vi "探头窗口-24-4列-网络版.vi"() -> ()   [LabVIEW 2017]
panel:
  in  "外部停止命令？":bool=TRUE
  out "引用-监测模式？":refnum<vi>
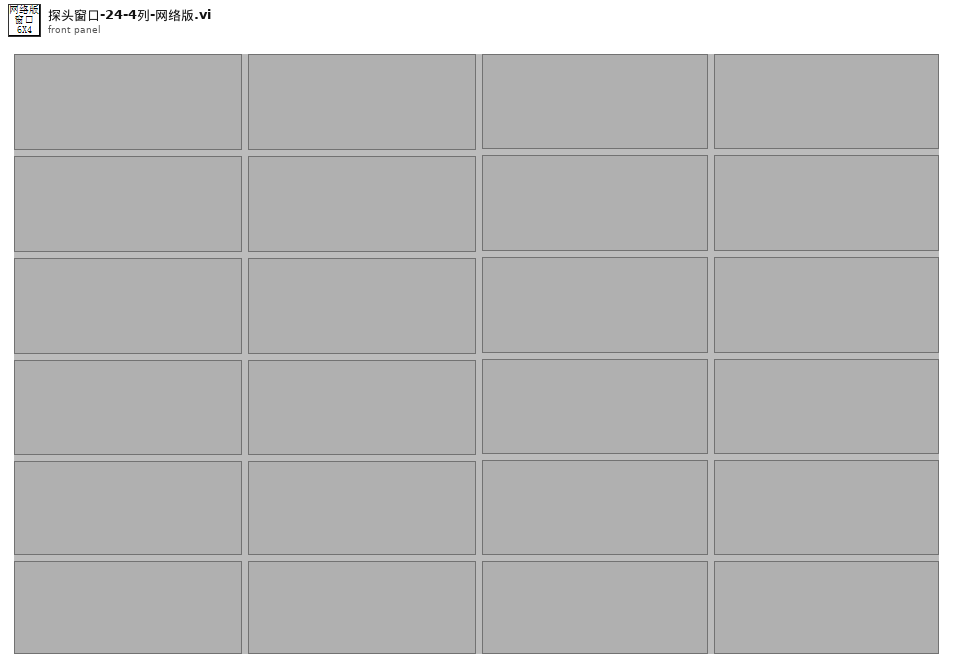
[diagram p1: front panel]
types:
  T1 = typedef "eventvkey.ctl" = enum16{"ASCII", "Enter", "Return", "Shift", "Ctrl", "Alt", "Cmd", "Opt", "Caps", "NumLock", "Clear", "Break", "Up", "Down", "Left", "Right", "Insert", "Delete", "Home", "End", "PageUp", "PageDown", "Escape", "Help", "Pause", "ScrollLock", "F1", "F2", "F3", "F4", "F5", "F6", "F7", "F8", "F9", "F10", "F11", "F12", "F13", "F14", "F15", "F16", "F17", "F18", "F19", "F20", "F21", "F22", "F23", "F24", "Play", "VolumeUp", "VolumeDown", "Mute", "Two Byte Char"}
  T2 = typedef "探头属性.ctl" = cluster{"探头地址与信息":T3, "测量值":T6, "限值":T7, "探头状态":T8, "累积记录":T9, "报警方式":T10}
  T3 = typedef "探测器信息.ctl" = cluster{"网络地址":string, "名称":string, "备注":string, "累积剂量":dbl, "累积限值":dbl, "硬件剂量率限值":T4, "剂量率限值1":dbl, "剂量率限值2":dbl, "报警方式":T5}
  T4 = typedef "探头剂量率限值选择.ctl" = enum16{"一级限值", "二级限值"}
  T5 = typedef "报警方式选择.ctl" = enum16{"常报警", "自动静音", "手动静音"}
  T6 = typedef "测量值.ctl" = cluster{"时间":timestamp, "数值":dbl}
  T7 = typedef "剂量率限值.ctl" = cluster{"限值1":dbl, "限值2":dbl, "探头限值":T4}
  T8 = typedef "探头状态.ctl" = enum16{"正常", "离线", "禁用", "一级报警", "二级报警", "累积报警"}
  T9 = typedef "单条累积记录.ctl" = cluster{"起始时间":timestamp, "结束时间":timestamp, "累积剂量":dbl}
  T10 = typedef "报警方式.ctl" = cluster{"报警方式":T5, "延迟计时":u16, "报警中？":bool}
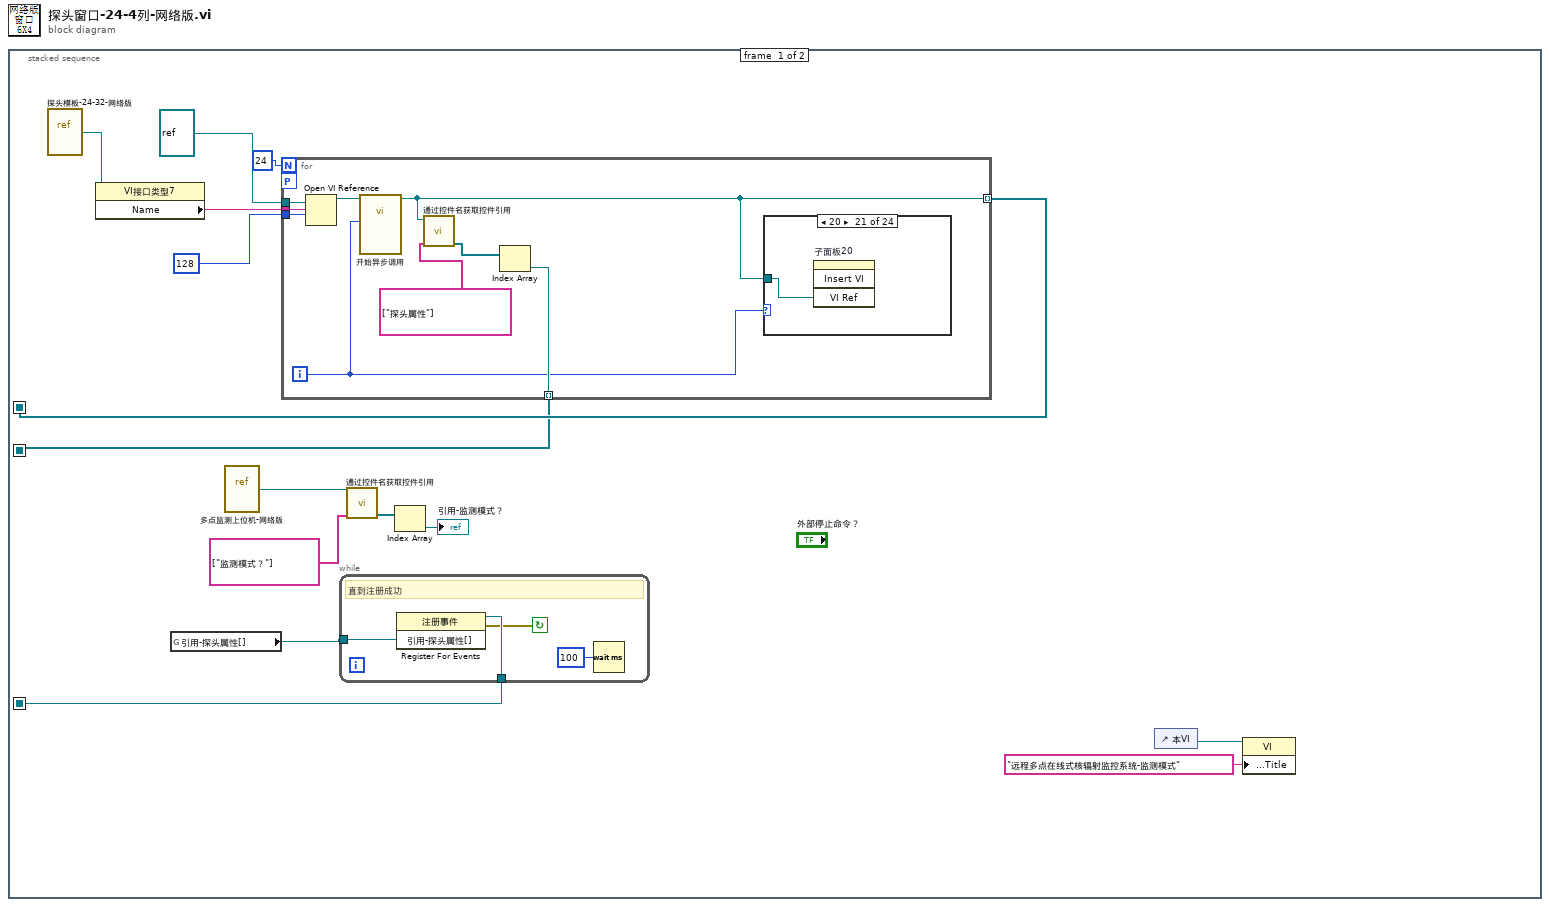
[diagram p0: block diagram]
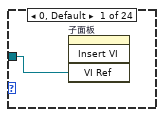
[diagram p2: hidden frame]
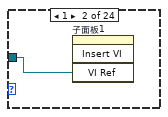
[diagram p3: hidden frame]
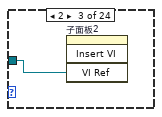
[diagram p4: hidden frame]
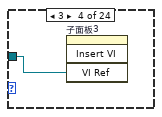
[diagram p5: hidden frame]
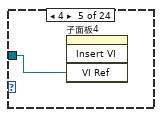
[diagram p6: hidden frame]
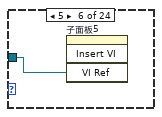
[diagram p7: hidden frame]
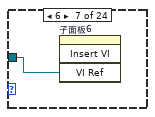
[diagram p8: hidden frame]
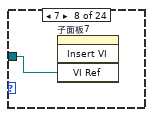
[diagram p9: hidden frame]
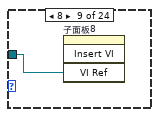
[diagram p10: hidden frame]
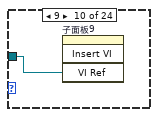
[diagram p11: hidden frame]
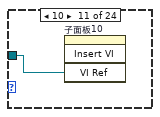
[diagram p12: hidden frame]
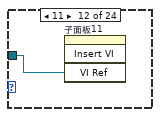
[diagram p13: hidden frame]
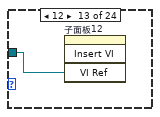
[diagram p14: hidden frame]
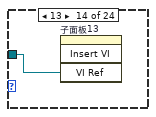
[diagram p15: hidden frame]
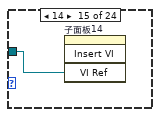
[diagram p16: hidden frame]
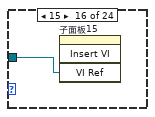
[diagram p17: hidden frame]
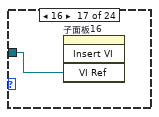
[diagram p18: hidden frame]
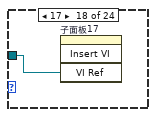
[diagram p19: hidden frame]
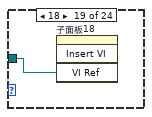
[diagram p20: hidden frame]
diagram:
  n1 = stacked-sequence {
    seq-local: [w11 _] -> [_ w55]
    seq-local: [w10 _] -> [_ w54]
    seq-local: [w1 _] -> [_ w53]
    frame #0 {
      n2 = vi-ref "探头模板-24-32-网络版.vi"() -> (w3:refnum<vi>)
      n3 = property class="VI接口类型7"(reference=w3) -> ("Name"=w15:string)  [unwired: 1 in, 2 out]
      n4 = global read "全局变量-35点监测.vi" "引用-探头属性[]"() -> (w2:refnum<vi>)
      n5 = vi-ref "多点监测上位机-网络版.vi"() -> (w6:refnum<vi>)
      n6 = for {
        N: 24 -> [_]
        tunnel: w15 -> [w28]
        tunnel: 128 ("选项") -> [w27]
        tunnel: refnum<vi> refnum ("类型说明符VI引用句柄（仅用于类型）") -> [w26]
        tunnel: [w21] -> w11 mode=indexing
        tunnel: [w23] -> w10 mode=indexing
        workers-P: _ -> [_]
        i -> [w20]
        n7 = Open VI Reference(type specifier VI Refnum (for type only)=w26, vi path=w28, options=w27) -> (vi reference=w22:refnum<vi>)  [unwired: 3 in, 1 out]
        n8 = call-by-ref "开始异步调用"(reference=w22, "探头序号"=w20) -> (reference out=w21:refnum<vi>)  [unwired: 12 in, 1 out]
        n9 = call "通过控件名获取控件引用.vi"("控件名数组"=string[] ["探头属性"], "VI引用"=w21) -> ("控件引用输出"=w25:refnum<vi>[])  [unwired: 7 in, 2 out]
        n10 = Index Array(array=w25) -> (element=w23:refnum<vi>)  [unwired: 1 in]
        n11 = case shown="20" w20 {
          tunnel: w21 -> [w29 w30 w31 w32 w33 w34 w35 w36 w37 w38 w39 w40 w41 w42 w43 w44 w45 w46 w47 w48 w49 w50 w51 w52]
          frame 0, Default {
            n12 = invoke on="子面板" class="子面板" method="Insert VI"("VI Ref"=w29) -> ()  [unwired: 3 in, 4 out]
          }
          frame 1 {
            n13 = invoke on="子面板1" class="SubPnl" method="Insert VI"("VI Ref"=w30) -> ()  [unwired: 3 in, 4 out]
          }
          frame 2 {
            n14 = invoke on="子面板2" class="SubPnl" method="Insert VI"("VI Ref"=w31) -> ()  [unwired: 3 in, 4 out]
          }
          frame 3 {
            n15 = invoke on="子面板3" class="SubPnl" method="Insert VI"("VI Ref"=w32) -> ()  [unwired: 3 in, 4 out]
          }
          frame 4 {
            n16 = invoke on="子面板4" class="SubPnl" method="Insert VI"("VI Ref"=w33) -> ()  [unwired: 3 in, 4 out]
          }
          frame 5 {
            n17 = invoke on="子面板5" class="SubPnl" method="Insert VI"("VI Ref"=w34) -> ()  [unwired: 3 in, 4 out]
          }
          frame 6 {
            n18 = invoke on="子面板6" class="SubPnl" method="Insert VI"("VI Ref"=w35) -> ()  [unwired: 3 in, 4 out]
          }
          frame 7 {
            n19 = invoke on="子面板7" class="SubPnl" method="Insert VI"("VI Ref"=w36) -> ()  [unwired: 3 in, 4 out]
          }
          frame 8 {
            n20 = invoke on="子面板8" class="SubPnl" method="Insert VI"("VI Ref"=w37) -> ()  [unwired: 3 in, 4 out]
          }
          frame 9 {
            n21 = invoke on="子面板9" class="SubPnl" method="Insert VI"("VI Ref"=w38) -> ()  [unwired: 3 in, 4 out]
          }
          frame 10 {
            n22 = invoke on="子面板10" class="SubPnl" method="Insert VI"("VI Ref"=w39) -> ()  [unwired: 3 in, 4 out]
          }
          frame 11 {
            n23 = invoke on="子面板11" class="SubPnl" method="Insert VI"("VI Ref"=w40) -> ()  [unwired: 3 in, 4 out]
          }
          frame 12 {
            n24 = invoke on="子面板12" class="SubPnl" method="Insert VI"("VI Ref"=w41) -> ()  [unwired: 3 in, 4 out]
          }
          frame 13 {
            n25 = invoke on="子面板13" class="SubPnl" method="Insert VI"("VI Ref"=w42) -> ()  [unwired: 3 in, 4 out]
          }
          frame 14 {
            n26 = invoke on="子面板14" class="SubPnl" method="Insert VI"("VI Ref"=w43) -> ()  [unwired: 3 in, 4 out]
          }
          frame 15 {
            n27 = invoke on="子面板15" class="SubPnl" method="Insert VI"("VI Ref"=w44) -> ()  [unwired: 3 in, 4 out]
          }
          frame 16 {
            n28 = invoke on="子面板16" class="SubPnl" method="Insert VI"("VI Ref"=w45) -> ()  [unwired: 3 in, 4 out]
          }
          frame 17 {
            n29 = invoke on="子面板17" class="SubPnl" method="Insert VI"("VI Ref"=w46) -> ()  [unwired: 3 in, 4 out]
          }
          frame 18 {
            n30 = invoke on="子面板18" class="SubPnl" method="Insert VI"("VI Ref"=w47) -> ()  [unwired: 3 in, 4 out]
          }
          frame 19 {
            n31 = invoke on="子面板19" class="SubPnl" method="Insert VI"("VI Ref"=w48) -> ()  [unwired: 3 in, 4 out]
          }
          frame 20 {
            n32 = invoke on="子面板20" class="SubPnl" method="Insert VI"("VI Ref"=w49) -> ()  [unwired: 3 in, 4 out]
          }
          frame 21 {
            n33 = invoke on="子面板21" class="SubPnl" method="Insert VI"("VI Ref"=w50) -> ()  [unwired: 3 in, 4 out]
          }
          frame 22 {
            n34 = invoke on="子面板22" class="SubPnl" method="Insert VI"("VI Ref"=w51) -> ()  [unwired: 3 in, 4 out]
          }
          frame 23 {
            n35 = invoke on="子面板23" class="SubPnl" method="Insert VI"("VI Ref"=w52) -> ()  [unwired: 3 in, 4 out]
          }
        }
      }
      n36 = while {
        tunnel: w2 -> [w19]
        tunnel: [w18] -> w1
        stop <- w17 continue-if-true
        # "直到注册成功"
        n37 = register-events(w19) -> (reference out=w18:refnum<event-registration>, error out=w17:errorcluster)  [unwired: 2 in]
        n38 = Wait (ms)(milliseconds to wait=u32 100 ("等待时间（毫秒）")) -> ()  [unwired: 1 out]
      }
      n39 = call "通过控件名获取控件引用.vi"("控件名数组"=string[] ["监测模式？"], "VI引用"=w6) -> ("控件引用输出"=w8:refnum<vi>[])  [unwired: 7 in, 2 out]
      n40 = Index Array(array=w8) -> (element=→"引用-监测模式？":refnum<vi>)  [unwired: 1 in]
      n41 = control-ref of="本VI"() -> (w5:refnum<vi>)
      n42 = property class="VI"(reference=w5, "Front Panel.Title"="远程多点在线式核辐射监控系统-监测模式" ("前面板窗口:标题")) -> ()  [unwired: 1 in, 2 out]
    }
    frame #1 {
      n43 = while {
        tunnel: w55 -> [w58]
        tunnel: w54 -> [w57]
        tunnel: w53 -> [w56]
        stop <- w59 stop-if-true
        n44 = event shown="[2] 键按下" {
          selector: w56 -> [_ _ _ w64 _]
          dyn-events: _ -> [_ _ _ _ _]
          timeout: _ -> [_ _ _ _ _]
          tunnel: [_ _ _ TRUE ("放弃？") _] -> w59
          tunnel: w58 -> [_ _ _ w66 _]
          tunnel: w57 -> [_ _ _ _ w83]
          event Timeout {
            n45 = event-data() -> ()  [unwired: 1 in, 3 out]
          }
          event Panel Close? {
            n46 = event-data() -> ()  [unwired: 1 in, 4 out]
            n47 = property on="外部停止命令？" class="Bool (严格)"("Val(Sgnl)"=FALSE ("值(信号)")) -> ()  [unwired: 2 in, 2 out]
            n48 = event-data("Discard?"=TRUE ("放弃？")) -> ()  [unwired: 1 in, 1 out]
          }
          event Key Down {
            n49 = event-data() -> ("VKey"=w62:T1)  [unwired: 1 in, 9 out]
            n50 = case shown="\"Enter\"" w62 {
              frame "ASCII", Default {
              }
              frame "Enter" {
                # "退出"
                n51 = property on="外部停止命令？" class="Bool (严格)"("Val(Sgnl)"=FALSE ("值(信号)")) -> ()  [unwired: 2 in, 2 out]
              }
            }
          }
          event "外部停止命令？": Value Change {
            n52 = event-data() -> ()  [unwired: 1 in, 6 out]
            n53 = flat-sequence {
              tunnel: w66 -> [w69]
              tunnel: [w69] -> w65
              tunnel: w64 -> [w68]
              tunnel: w65 -> [w76]
              frame #0 {
                n54 = Unregister For Events(event registration refnum=w68) -> ()  [unwired: 1 in, 1 out]
              }
              frame #1 {
                w75 = FALSE  # F
                n55 = local read "引用-监测模式？"() -> (w74:refnum<vi>)
                n56 = for {
                  tunnel: w76 -> [w81] mode=indexing
                  workers-P: _ -> [_]
                  tunnel: [w77] -> w71
                  n57 = invoke class="VI (严格)" method="Abort VI"(reference=w81) -> (reference out=w79:refnum<vi>, error out=w80:errorcluster)  [unwired: 2 in, 1 out]
                  n58 = Close Reference(reference=w79, error in (no error)=w80) -> (error out=w78:errorcluster)
                  n59 = call <vilib>:"Clear Errors.vi"("error in (no error)"=w78) -> ("error out"=w77:errorcluster)  [unwired: 5 in, 1 out]
                }
                n60 = control-ref of="本VI"() -> (w73:refnum<vi>)
                n61 = property class="Ctl"(reference=w74, error in=w71, "Val(Sgnl)"=w75) -> (error out=w70:errorcluster)  [unwired: 1 out]
                n62 = invoke class="VI" method="FP.Close"(reference=w73, error in=w70) -> (error out=w72:errorcluster)  [unwired: 1 in, 2 out]
                n63 = call <vilib>:"Clear Errors.vi"("error in (no error)"=w72) -> ()  [unwired: 5 in, 2 out]
              }
            }
          }
          event Value Change {
            n64 = event-data() -> ("NewVal"=w82:T2[])  [unwired: 1 in, 5 out]
            n65 = for {
              workers-P: _ -> [_]
              tunnel: w83 -> [w85] mode=indexing
              tunnel: w82 -> [w84] mode=indexing
              # "各个“探头属性”赋值（信号）"
              n66 = property class="Ctl"(reference=w85, "Val(Sgnl)"=w84) -> ()  [unwired: 1 in, 2 out]
            }
          }
        }
      }
    }
  }
